vi "VisionGetTarget.vi"(8 "LimelightActivate":bool, 9 "Camera Pitch [deg.]":dbl, 10 "Camera Height[in.]":dbl=30.0, 11 "Limelight name":string="limelight") -> (3 "VisionTarget":T1)   [LabVIEW 2019]
uses:
  TypeDefs/VisionTarget.ctl
  ArgosLib/Signal Processing/TypeDefs/EdgeDetector_Type.ctl
  <vilib>/Rock Robotics/Network Tables/NT Read Number.vi
  <vilib>/Rock Robotics/Network Tables/NT Read Numeric Array.vi
  <vilib>/Rock Robotics/Network Tables/NT Write Number.vi
  TypeDefs/VisionPipeline.ctl
  ArgosLib/ArgosLib.lvlib
panel:
  out "tcorny":dbl[](array[numeric])
  out "tcornx":dbl[](array[numeric])
  out "FieldCentricAngleToTarget":dbl
  out "thor":dbl
  out "tvert":dbl
  out "ar":dbl
  out "Target Found?":bool
  out "raw ty":dbl
  out "TimeToAcquireTarget(ms)":u32
  out "Distance (Area-T_vertical)[In.]":dbl
  out "tx":dbl
  out "Distance (Angle.)[In.]":dbl
  in  "Target Height[in.]":dbl=100.0
  out "ta":dbl
  out "tvert":dbl
  out "thor":dbl
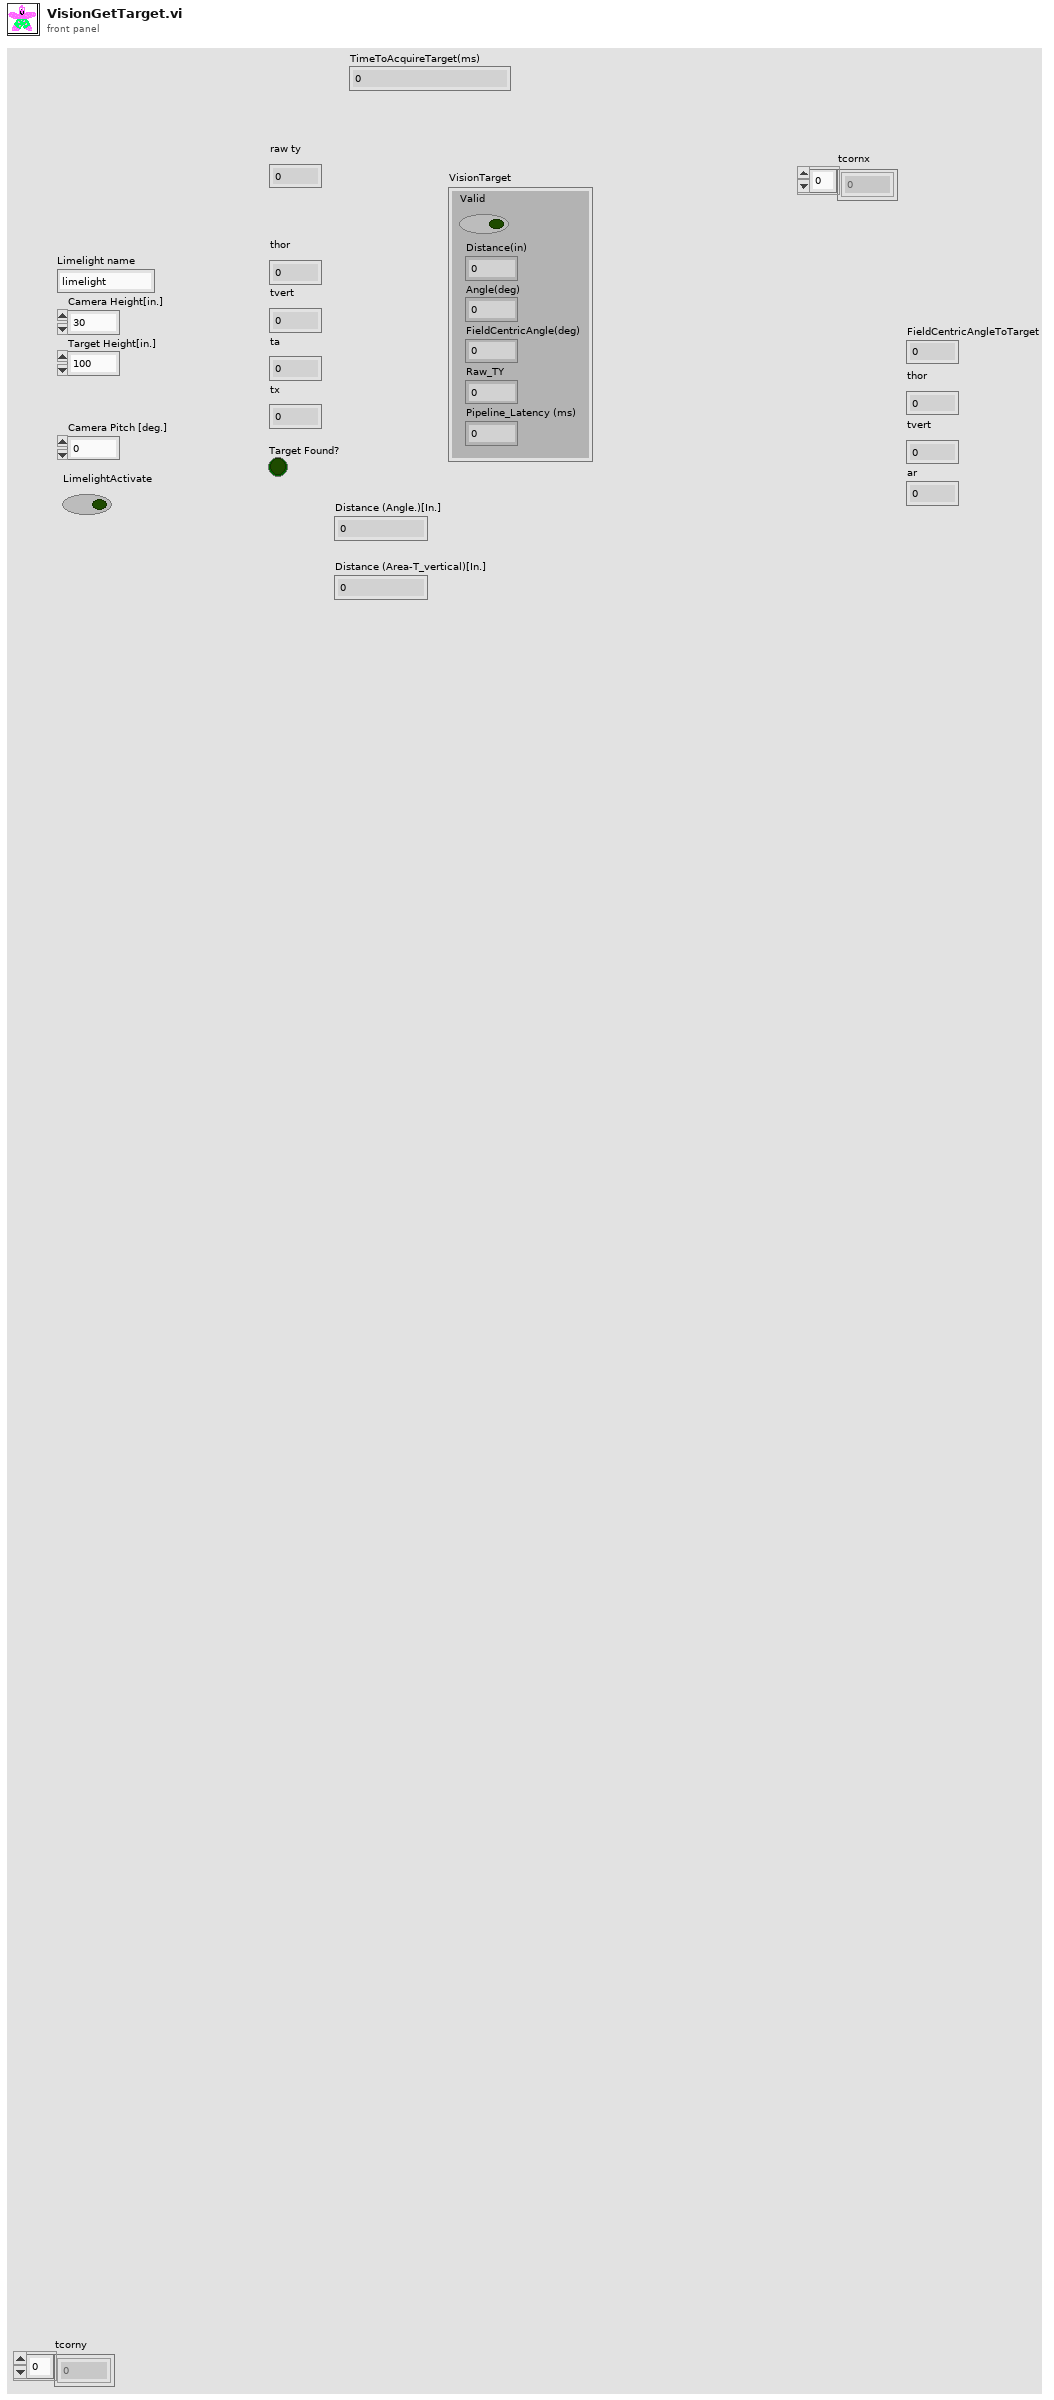
[diagram p1: front panel]
types:
  T1 = typedef "VisionTarget.ctl" = cluster{"Valid":bool, "Distance(in)":dbl, "Angle(deg)":dbl, "FieldCentricAngle(deg)":dbl, "Raw_TY":dbl, "Pipeline_Latency (ms)":dbl}
  T2 = typedef "ArgosLib.lvlib/EdgeDetector_Type.ctl" = enum16{"RisingEdge", "FallingEdge", "Both"}
  T3 = typedef "VisionPipeline.ctl" = enum16{"LEDOff", "NoZoom", "Zoom2x", "Zoom3x"}
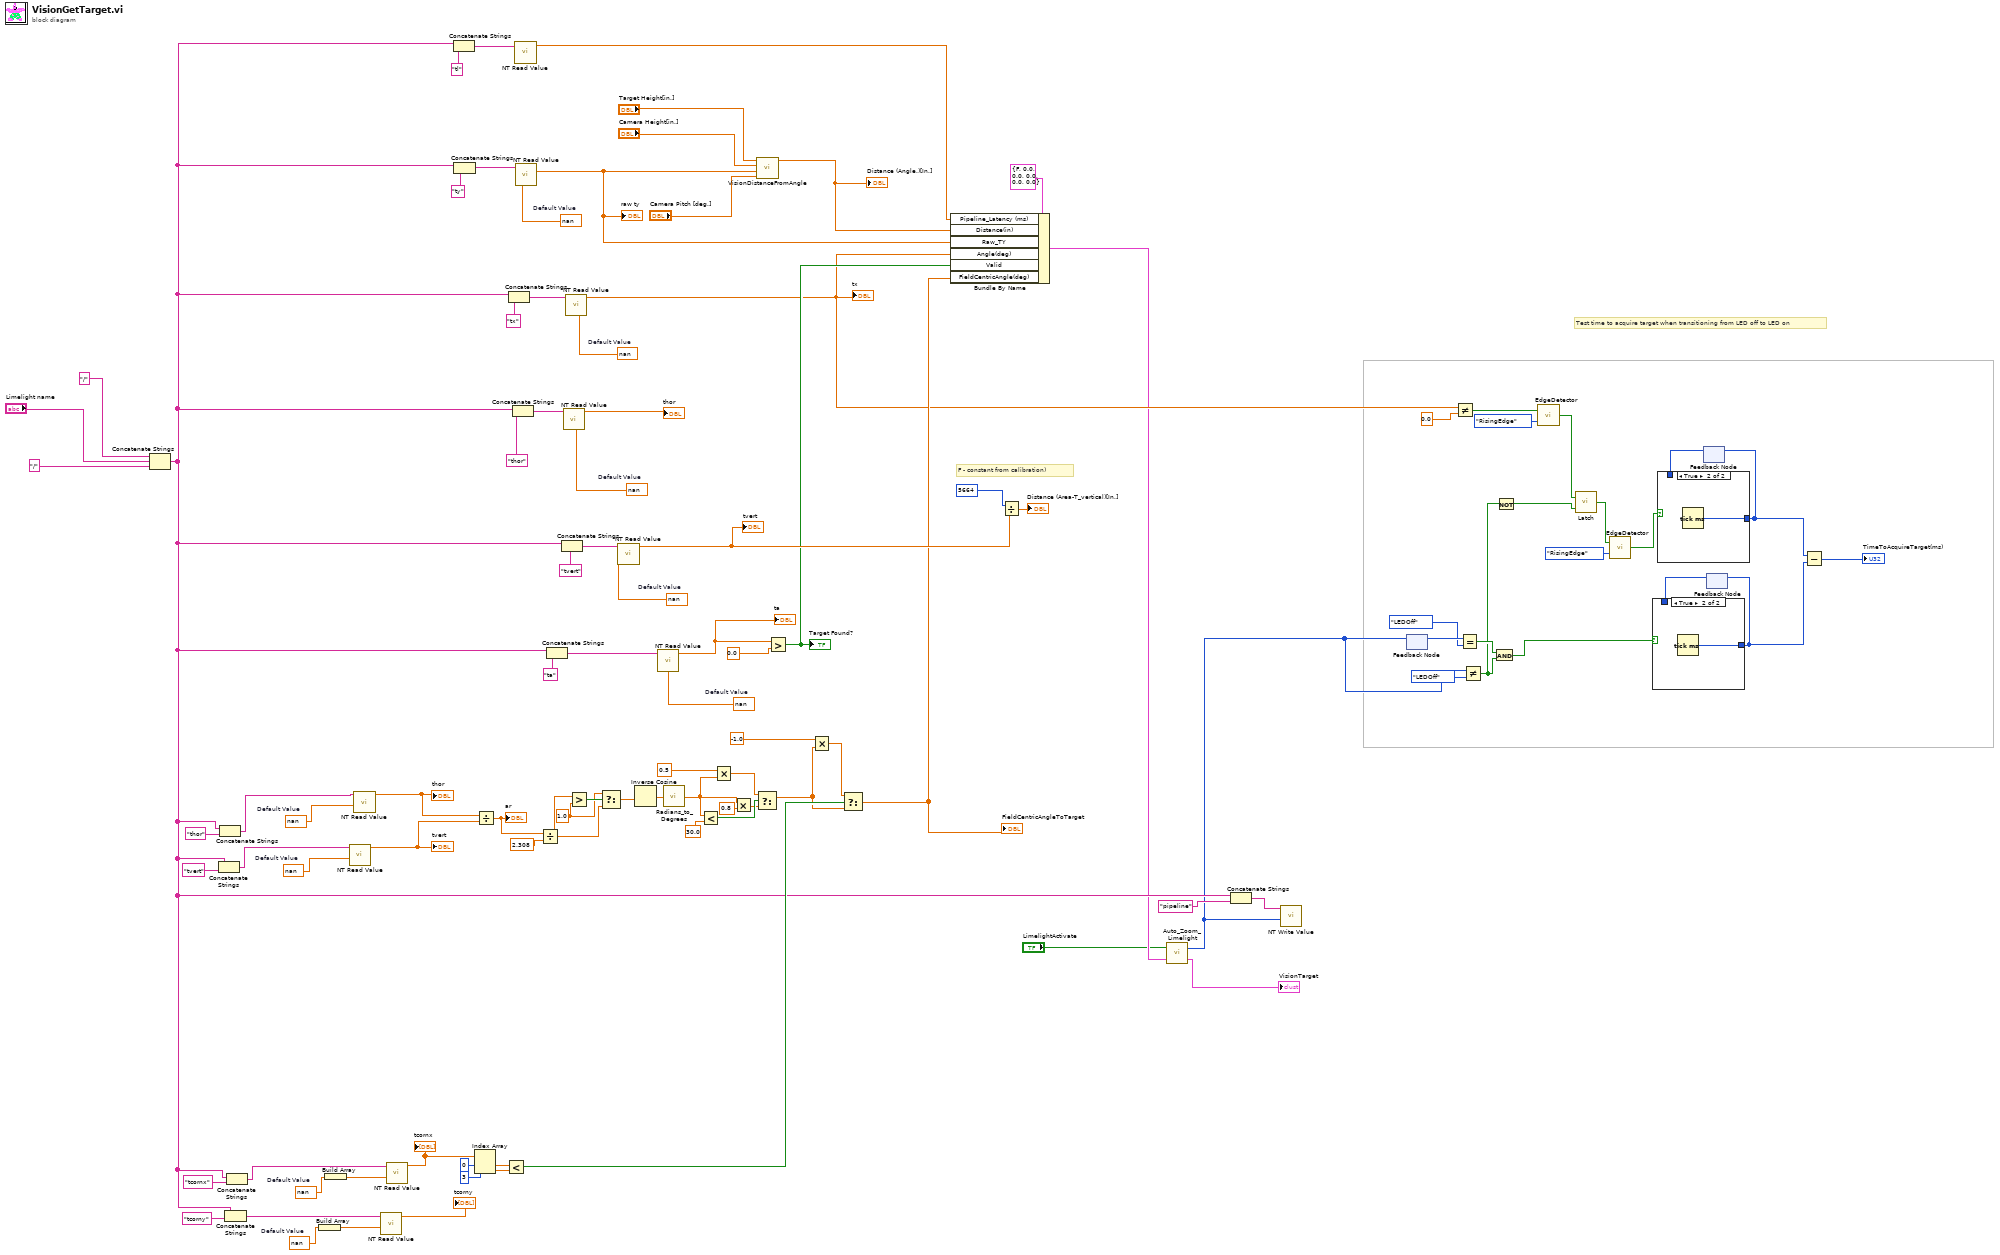
[diagram p0: block diagram]
diagram:
  w23 = nan  # Default Value
  w26 = nan  # Default Value
  w38 = 1.0 ("y")
  w50 = nan  # Default Value
  w49 = nan  # Default Value
  w84 = nan  # Default Value
  w102 = nan  # Default Value
  w100 = nan  # Default Value
  w99 = nan  # Default Value
  w98 = nan  # Default Value
  # "Test time to acquire target when transitioning from LED off to LED on"
  # "F - constant from calibration)"
  n1 = Concatenate Strings("/" ("string"), "Limelight name", "/" ("string")) -> (w7:string)
  n2 = Concatenate Strings(w7, "tvert" ("Name")) -> (w48:string)
  n3 = Concatenate Strings(w7, "thor" ("Name")) -> (w45:string)
  n4 = Concatenate Strings(w7, "tcorny" ("Name")) -> (w21:string)
  n5 = Concatenate Strings(w7, "tcornx" ("Name")) -> (w27:string)
  n6 = Build Array(w23) -> (w22:dbl[])
  n7 = Build Array(w26) -> (w25:dbl[])
  n8 = call-poly <vilib>:"NT Read Value.vi"("Default Value"=w50, "Name"=w48) -> ("Numeric"=w51:dbl)  [unwired: 8 in, 1 out]
  "tvert" <- w51
  n9 = call-poly <vilib>:"NT Read Value.vi"("Default Value"=w49, "Name"=w45) -> ("Numeric"=w44:dbl)  [unwired: 8 in, 1 out]
  "thor" <- w44
  n10 = call-poly <vilib>:"NT Read Value.vi"("Default Value"=w22, "Name"=w21) -> ("Numeric Array"=→"tcorny":dbl[])  [unwired: 8 in, 1 out]
  n11 = call-poly <vilib>:"NT Read Value.vi"("Default Value"=w25, "Name"=w27) -> ("Numeric Array"=w20:dbl[])  [unwired: 8 in, 1 out]
  "tcornx" <- w20
  n12 = Concatenate Strings(w7, "tl" ("string")) -> (w10:string)
  n13 = Concatenate Strings(w7, "ty" ("Name")) -> (w83:string)
  n14 = Index Array(array=w20, index #1=0 ("index"), index #2=3 ("index")) -> (element #1=w16:dbl, element #2=w17:dbl)
  n15 = Divide(x=w44, y=w51) -> (x/y=w43:dbl)
  "ar" <- w43
  n16 = Less?(x=w16, y=w17) -> (x < y?=w15:bool)
  n17 = Concatenate Strings(w7, "tx" ("Name")) -> (w86:string)
  n18 = Concatenate Strings(w7, "thor" ("Name")) -> (w93:string)
  n19 = call-poly <vilib>:"NT Read Value.vi"("Name"=w10) -> ("Numeric"=w8:dbl)  [unwired: 9 in, 1 out]
  n20 = call-poly <vilib>:"NT Read Value.vi"("Default Value"=w98, "Name"=w83) -> ("Numeric"=w5:dbl)  [unwired: 8 in, 1 out]
  "raw ty" <- w5
  n21 = Divide(x=w43, y=2.308) -> (x/y=w39:dbl)
  n22 = Concatenate Strings(w7, "ta" ("Name")) -> (w89:string)
  n23 = Concatenate Strings(w7, "tvert" ("Name")) -> (w91:string)
  n24 = call-poly <vilib>:"NT Read Value.vi"("Default Value"=w99, "Name"=w93) -> ("Numeric"=→"thor":dbl)  [unwired: 8 in, 1 out]
  n25 = call-poly <vilib>:"NT Read Value.vi"("Default Value"=w84, "Name"=w86) -> ("Numeric"=w6:dbl)  [unwired: 8 in, 1 out]
  "tx" <- w6
  n26 = Greater?(x=w39, y=w38) -> (0:w40:bool)
  n27 = Select(t=w38, s=w40, f=w39) -> (s? t:f=w37:dbl)
  n28 = call-poly <vilib>:"NT Read Value.vi"("Default Value"=w100, "Name"=w91) -> ("Numeric"=w80:dbl)  [unwired: 8 in, 1 out]
  "tvert" <- w80
  n29 = Inverse Cosine(1:w37) -> (0:w41:dbl)
  n30 = call-poly <vilib>:"NT Read Value.vi"("Default Value"=w102, "Name"=w89) -> ("Numeric"=w57:dbl)  [unwired: 8 in, 1 out]
  "ta" <- w57
  n31 = call "Radians_to_Degrees.vi"("Radians"=w41) -> ("Degrees"=w32:dbl)
  n32 = Less?(x=w32, y=30.0) -> (x < y?=w35:bool)
  n33 = Multiply(x=0.5, y=w32) -> (x*y=w33:dbl)
  n34 = Multiply(x=w32, y=0.8) -> (x*y=w30:dbl)
  n35 = call "VisionDistanceFromAngle.vi"("PitchOffset(deg)"="Camera Pitch [deg.]", "Ty"=w5, "Camera Height[in.]"="Camera Height[in.]", "Target Height[in.]"="Target Height[in.]") -> ("Dist. From Target[in.]"=w54:dbl)  [unwired: 7 in]
  "Distance (Angle.)[In.]" <- w54
  n36 = Select(t=w33, s=w35, f=w30) -> (s? t:f=w13:dbl)
  n37 = Greater?(x=w57, y=0.0) -> (0:w53:bool)
  "Target Found?" <- w53
  n38 = Multiply(x=-1.0, y=w13) -> (x*y=w14:dbl)
  n39 = Select(t=w14, s=w15, f=w13) -> (s? t:f=w11:dbl)
  "FieldCentricAngleToTarget" <- w11
  n40 = Bundle By Name(cluster=T1 {"Valid"=FALSE, "Distance(in)"=0.0, "Angle(deg)"=0.0, "FieldCentricAngle(deg)"=0.0, "Raw_TY"=0.0, "Pipeline_Latency (ms)"=0.0} ("VisionTarget"), "Pipeline_Latency (ms)"=w8, "Distance(in)"=w54, "Raw_TY"=w5, "Angle(deg)"=w6, "Valid"=w53, "FieldCentricAngle(deg)"=w11) -> (w2:T1)
  n41 = Divide(x=5664, y=w80) -> (x/y=→"Distance (Area-T_vertical)[In.]":dbl)
  n42 = call "Auto_Zoom_Limelight.vi"("VisionTarget"=w2, "LimeLightActivate"="LimelightActivate") -> ("VisionTarget Out"=→"VisionTarget":T1, "Zoom_Indicator"=w4:T3)
  n43 = Concatenate Strings(w7, "pipeline" ("Name")) -> (w58:string)
  n44 = call-poly <vilib>:"NT Write Value.vi"("Numeric"=w4, "Name"=w58) -> ()  [unwired: 9 in, 1 out]
  n45 = feedback-in #1(w4) -> ()
  n46 = feedback #1() -> (w78:T3)  [unwired: 1 in]
  n47 = Not Equal?(x=w6, y=0.0) -> (x != y?=w67:bool)
  n48 = Equal?(x=w78, y=VisionPipeline."LEDOff") -> (x = y?=w75:bool)
  n49 = Not Equal?(x=w4, y=VisionPipeline."LEDOff") -> (x != y?=w61:bool)
  n50 = And(x=w75, y=w61) -> (x .and. y?=w73:bool)
  n51 = Not(x=w61) -> (.not. x?=w60:bool)
  n52 = call "EdgeDetector.vi"("DetectorType"=EdgeDetector_Type."RisingEdge", "Input"=w67) -> ("Edge"=w65:bool)
  n53 = call "Latch.vi"("Reset"=w60, "Input"=w65) -> ("LatchOut"=w63:bool)
  n54 = call "EdgeDetector.vi"("DetectorType"=EdgeDetector_Type."RisingEdge", "Input"=w63) -> ("Edge"=w62:bool)
  n55 = feedback #2() -> (w71:u32)  [unwired: 1 in]
  n56 = case shown="True" w62 {
    tunnel: [w103 w104] -> w70
    tunnel: w71 -> [w103 _]
    frame False {
    }
    frame True {
      n57 = Tick Count (ms)() -> (millisecond timer value=w104:u32)
    }
  }
  n58 = feedback-in #2(w70) -> ()
  n59 = feedback #3() -> (w74:u32)  [unwired: 1 in]
  n60 = case shown="True" w73 {
    tunnel: [w105 w106] -> w69
    tunnel: w74 -> [w105 _]
    frame False {
    }
    frame True {
      n61 = Tick Count (ms)() -> (millisecond timer value=w106:u32)
    }
  }
  n62 = feedback-in #3(w69) -> ()
  n63 = Subtract(x=w70, y=w69) -> (x-y=→"TimeToAcquireTarget(ms)":u32)
